vi "Event Handle Loop_Set Button Attribute.vi"(8 "error in (no error)":errorcluster, 10 "Button Attribute":T1, 11 "QMenu Class in":refnum<class "QMenu Class.lvclass">) -> (0 "error out":errorcluster, 3 "QMenu Class out":refnum<class "QMenu Class.lvclass">)   [LabVIEW 2020, in "QTab.lvlib" / "QMenu Class.lvclass"]
uses:
  QMenu Class.lvclass
  Button Attribute.ctl
  QMenu Class.lvclass/QMenu Class.ctl
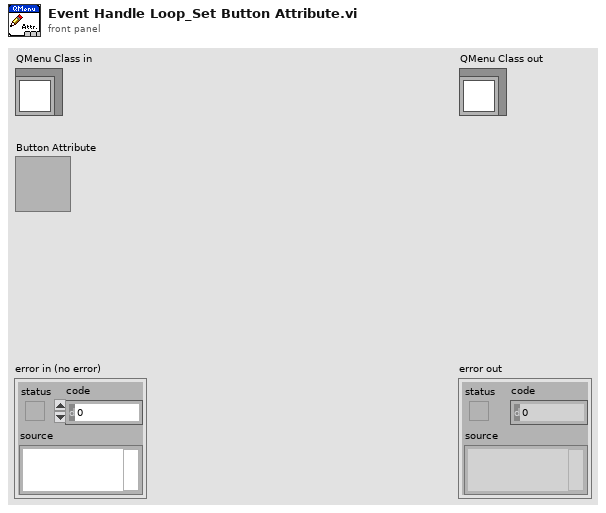
[diagram p1: front panel]
types:
  T1 = typedef "QTab.lvlib/QMenu Class.lvclass/Button Attribute.ctl" = cluster{"Label":string, "Button Text":string, "Closable":bool, "Draggable":bool}
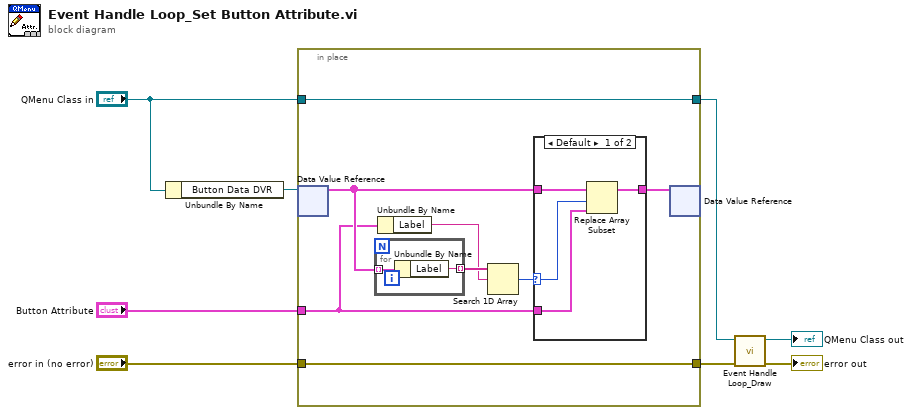
[diagram p0: block diagram]
diagram:
  n1 = Unbundle By Name("QMenu Class in") -> ("Button Data DVR"=w8:refnum<data-value>)
  n2 = in-place {
    in-place-border: "QMenu Class in" -> [w16]
    in-place-border: [w16] -> w3
    in-place-border: "error in (no error)" -> [w15]
    in-place-border: [w15] -> w4
    in-place-border: "Button Attribute" -> [w10]
    n3 = in-place-dvr #1(w8) -> (w11:T1[])  [unwired: 1 out]
    n4 = for {
      tunnel: w11 -> [w23] mode=indexing
      tunnel: [w22] -> w14 mode=indexing
      n5 = Unbundle By Name(w23) -> ("Label"=w22:string)
    }
    n6 = Unbundle By Name(w10) -> ("Label"=w13:string)
    n7 = Search 1D Array(1D array=w14, element=w13) -> (index of element=w12:i32)  [unwired: 1 in]
    n8 = case shown="Default" w12 {
      selector: w12 -> [w18 _]
      tunnel: w11 -> [w20 w21]
      tunnel: w10 -> [w17 _]
      tunnel: [w19 w21] -> w9
      frame Default {
        n9 = Replace Array Subset(array=w20, new element=w17, index=w18) -> (w19:T1[])
      }
      frame -1 {
      }
    }
    n10 = in-place-dvr #1(w9) -> ()  [unwired: 2 out]
  }
  n11 = call "Event Handle Loop_Draw.vi"("error in (no error)"=w4, "QMenu Class in"=w3) -> ("error out"=→"error out":errorcluster, "QMenu Class out"=→"QMenu Class out":refnum<class "QMenu Class.lvclass">)  [unwired: 8 in]
